vi "SDCP SMF Receiver and Transmitter - Trace File.vi"(2 "error in (no error)":errorcluster, 3 "Trace file path":path) -> (0 "error out":errorcluster)   [LabVIEW 2020]
uses:
  <vilib>/Utility/file.llb/Write Delimited Spreadsheet (string).vi
  <vilib>/Utility/file.llb/Write Delimited Spreadsheet (DBL).vi
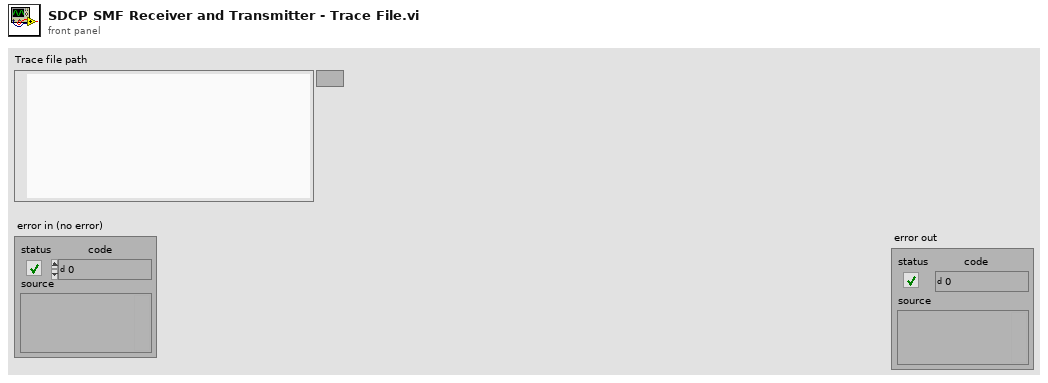
[diagram p1: front panel]
types:
  T1 = typedef "SDCP SMF Receiver and Transmitter - Notifier and Queues.ctl" = cluster{"Trace Queue":refnum<queue>, "Tx - Log Table Queue":refnum<queue>, "Tx - User Queue":refnum<queue>, "Rx - Log Table Queue":refnum<queue>, "Rx - User Queue":refnum<queue>, "Log status Notifier":refnum<notifier>, "Plot Queue":refnum<queue>}
  T2 = typedef "SDCP SMF logger - SMF with timestamp.ctl" = cluster{"Bytes":u8[], "Checksum":bool, "Time (ms)":u32, "Tx/Rx":string}
  T3 = enum16{"open", "replace", "create", "open or create", "replace or create", "replace or create with confirmation"}
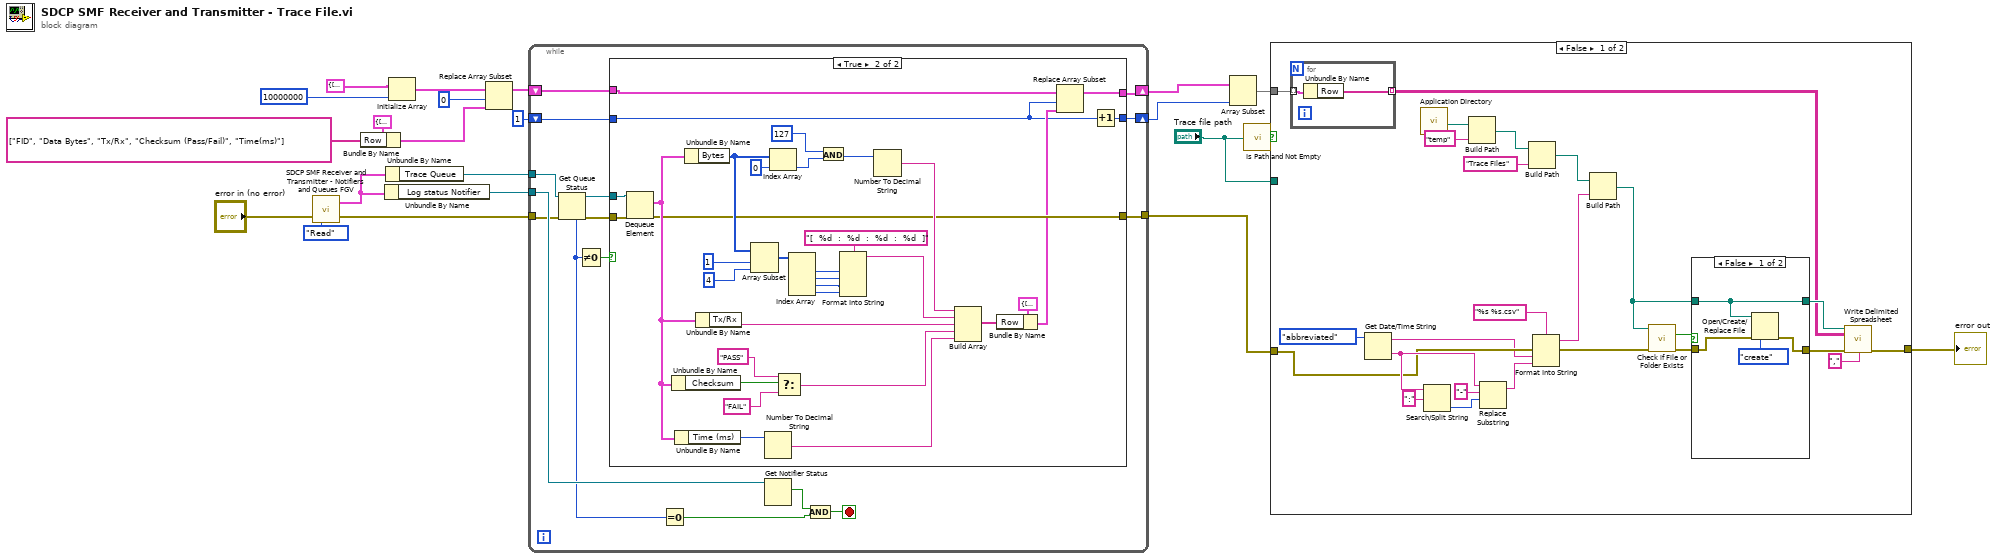
[diagram p0: block diagram]
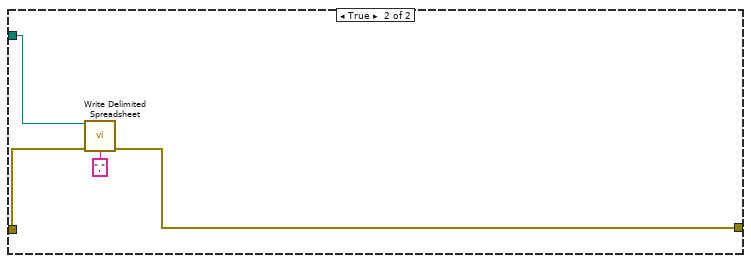
[diagram p3: hidden frame]
diagram:
  n1 = call "SDCP SMF Receiver and Transmitter - Notifiers and Queues FGV.vi"("error in (no error)"="error in (no error)", "Command"=enum16{"Initialize", "Read", "Deinitialize"}."Read") -> ("error out"=w20:errorcluster, "Output"=w19:T1)
  n2 = Bundle By Name(cluster=cluster{"Row":string[]} {"Row"=["", "", "", "", ""]}, "Row"=string[] ["FID", "Data Bytes", "Tx/Rx", "Checksum (Pass/Fail)", "Time(ms)"]) -> (w6:cluster{"Row":string[]})
  n3 = Unbundle By Name(w19) -> ("Log status Notifier"=w18:refnum<notifier>)
  n4 = Unbundle By Name(w19) -> ("Trace Queue"=w17:refnum<queue>)
  n5 = Initialize Array(cluster{"Row":string[]} {"Row"=["", "", "", "", ""]}, 10000000 ("dimension size")) -> (w10:cluster{"Row":string[]}[])
  n6 = Replace Array Subset(array=w10, new element=w6, index=0) -> (w5:cluster{"Row":string[]}[])
  n7 = while {
    tunnel: w20 -> [w34]
    tunnel: w18 -> [w37]
    shift-right: [w23] -> w1
    shift-left: w5 -> [w36]
    tunnel: w17 -> [w32]
    tunnel: [w35] -> w15
    shift-right: [w25] -> w2
    shift-left: 1 -> [w26]
    stop <- w28 stop-if-true
    n8 = Get Queue Status(queue=w32, error in (no error)=w34) -> (queue out=w31:refnum<queue>, error out=w33:errorcluster, # elements in queue=w27:i32)  [unwired: 1 in, 5 out]
    n9 = Not Equal To 0?(x=w27) -> (x != 0?=w30:bool)
    n10 = case shown="True" w30 {
      tunnel: w36 -> [w40 w45]
      tunnel: [w40 w44] -> w23
      tunnel: [w39 w50] -> w35
      tunnel: w33 -> [w39 w49]
      tunnel: w31 -> [_ w48]
      tunnel: w26 -> [w38 w42]
      tunnel: [w38 w41] -> w25
      frame False {
      }
      frame True {
        n11 = Dequeue Element(queue=w48, error in (no error)=w49) -> (element=w57:T2, error out=w50:errorcluster)  [unwired: 1 in, 2 out]
        n12 = Unbundle By Name(w57) -> ("Checksum"=w60:bool)
        n13 = Unbundle By Name(w57) -> ("Time (ms)"=w56:u32)
        n14 = Unbundle By Name(w57) -> ("Bytes"=w69:u8[])
        n15 = Unbundle By Name(w57) -> ("Tx/Rx"=w53:string)
        n16 = Array Subset(array=w69, index=1, length=4) -> (w66:u8[])
        n17 = Number To Decimal String(number=w56) -> (decimal integer string=w51:string)  [unwired: 1 in]
        n18 = Index Array(array=w69, index=0) -> (element=w72:u8)
        n19 = Select(t="PASS", s=w60, f="FAIL") -> (s? t:f=w52:string)
        n20 = Index Array(array=w66) -> (element #1=w64:u8, element #2=w63:u8, element #3=w62:u8, element #4=w61:u8)  [unwired: 4 in]
        n21 = And(x=u8 127, y=w72) -> (x .and. y?=w70:u8)
        n22 = Format Into String(format string="[  %d  :  %d  :  %d  :  %d  ]", w64, w63, w62, w61) -> (resulting string=w54:string)  [unwired: 2 in, 1 out]
        n23 = Number To Decimal String(number=w70) -> (decimal integer string=w55:string)  [unwired: 1 in]
        n24 = Build Array(w55, w54, w53, w52, w51) -> (w47:string[])
        n25 = Bundle By Name(cluster=cluster{"Row":string[]} {"Row"=["", "", "", "", ""]}, "Row"=w47) -> (w43:cluster{"Row":string[]})
        n26 = Replace Array Subset(array=w45, new element=w43, index=w42) -> (w44:cluster{"Row":string[]}[])
        n27 = Increment(x=w42) -> (x+1=w41:i32)
      }
    }
    n28 = Equal To 0?(x=w27) -> (x = 0?=w24:bool)
    n29 = Get Notifier Status(notifier=w37) -> (current notification=w29:bool)  [unwired: 1 in, 4 out]
    n30 = And(x=w29, y=w24) -> (x .and. y?=w28:bool)
  }
  n31 = Array Subset(array=w1, length=w2) -> (w3:cluster{"Row":string[]}[])  [unwired: 1 in]
  n32 = call <vilib>:"Is Path and Not Empty.vi"("path"="Trace file path") -> ("Is Path and Not Empty?"=w16:bool)  [unwired: 4 in]
  n33 = case shown="False" w16 {
    tunnel: w15 -> [w90 w109]
    tunnel: w3 -> [w75 _]
    tunnel: "Trace file path" -> [_ w108]
    tunnel: [w81 w107] -> w13
    frame False {
      n34 = for {
        tunnel: w75 -> [w100] mode=indexing
        tunnel: [w99] -> w74 mode=indexing
        n35 = Unbundle By Name(w100) -> ("Row"=w99:string[])
      }
      n36 = Get Date/Time String(date format (0)=enum16{"short", "long", "abbreviated"}."abbreviated") -> (date string=w77:string, time string=w94:string)  [unwired: 2 in]
      n37 = call <vilib>:"Application Directory.vi"() -> ("Application Directory"=w98:path)
      n38 = Search/Split String(string=w94, search string/char (-)=":") -> (offset of match=w78:i32)  [unwired: 1 in, 2 out]
      n39 = Build Path(base path=w98, name or relative path="temp") -> (appended path=w85:path)
      n40 = Replace Substring(3:w78, 4:"-" ("substring (\"\")"), 5:w94) -> (1:w76:string)  [unwired: 1 in, 1 out]
      n41 = Build Path(base path=w85, name or relative path="Trace Files") -> (appended path=w83:path)
      n42 = Format Into String(format string="%s %s.csv", error in=w90, w77, w76) -> (resulting string=w91:string, error out=w89:errorcluster)  [unwired: 1 in]
      n43 = Build Path(base path=w83, name or relative path=w91) -> (appended path=w86:path)
      n44 = call <vilib>:"Check if File or Folder Exists.vi"("error in (no error)"=w89, "path"=w86) -> ("error out"=w87:errorcluster, "file or folder exists?"=w88:bool)  [unwired: 7 in, 1 out]
      n45 = case shown="False" w88 {
        tunnel: w87 -> [w104 w105]
        tunnel: w86 -> [w102 w106]
        tunnel: [w102 w106] -> w80
        tunnel: [w103 w105] -> w82
        frame False {
          n46 = Open/Create/Replace File(file path (use dialog)=w102, error in=w104, operation (0:open)=T3."create") -> (error out=w103:errorcluster)  [unwired: 3 in, 2 out]
        }
        frame True {
        }
      }
      n47 = call-poly <vilib>:"Write Delimited Spreadsheet.vi"("file path (dialog if empty)"=w80, "2D data"=w74, "error in (no error)"=w82, "delimiter (\\t)"="," ("delimiter (\\t)")) -> ("error out"=w81:errorcluster)  [unwired: 10 in, 1 out]
    }
    frame True {
      n48 = call-poly <vilib>:"Write Delimited Spreadsheet.vi"("file path (dialog if empty)"=w108, "error in (no error)"=w109, "delimiter (\\t)"="," ("delimiter (\\t)")) -> ("error out"=w107:errorcluster)  [unwired: 11 in, 1 out]
    }
  }
  "error out" <- w13
